vi "Buffer Num Readings.vi"(8 "error in (no error)":errorcluster, 9 "Buffer Name":string, 11 "VISA resource name":refnum<visa-resource-name>) -> (0 "error out":errorcluster, 1 "Number of Readings in Buffer":u32, 3 "VISA resource name out":refnum<visa-resource-name>, 4 "Command String":string)   [LabVIEW 2012, in "Keithley 2600 Series.lvlib"]
doc: "This VI queries the number of readings in the selected buffer.\n\n<b>Functions and Attributes Used</b>\n<buffername>.n"
uses:
  Keithley 2600 Series.lvlib
  Private/GlobalVariables.vi
panel:
  # "(c) 2008 Keithley Instruments, Inc.  ALL RIGHTS RESERVED."
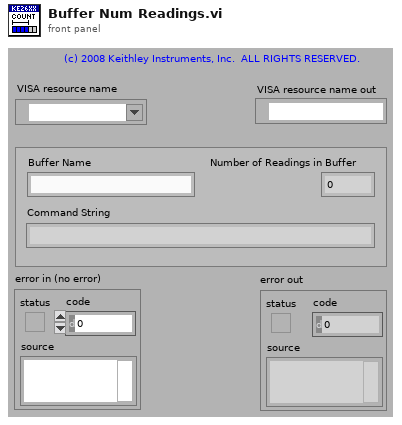
[diagram p1: front panel]
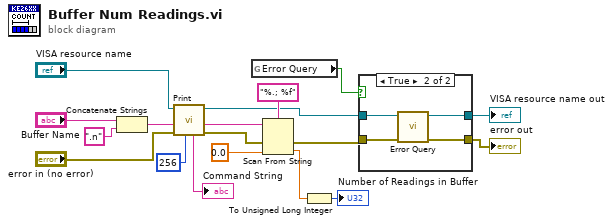
[diagram p0: block diagram]
diagram:
  n1 = Concatenate Strings("Buffer Name", ".n" ("string")) -> (w8:string)
  n2 = call "Print.vi"("Byte Count (1024)"=u32 256, "error in (no error)"="error in (no error)", "Input"=w8, "VISA resource name"="VISA resource name") -> ("error out"=w2:errorcluster, "Output"=w3:string, "VISA resource name out"=w1:refnum<visa-resource-name>, "Command String"=→"Command String":string)  [unwired: 1 in, 3 out]
  n3 = global read "GlobalVariables.vi" "Error Query"() -> (w14:bool)
  n4 = Scan From String(format string="%.; %f", input string=w3, error in=w2, default 1=0.0 ("default value 1")) -> (error out=w13:errorcluster, output 1=w15:dbl)  [unwired: 1 in, 2 out]
  n5 = To Unsigned Long Integer(number=w15) -> (unsigned 32bit integer=→"Number of Readings in Buffer":u32)
  n6 = case shown="True" w14 {
    tunnel: w13 -> [w20 w24]
    tunnel: [w19 w23] -> w12
    tunnel: [w20 w22] -> w11
    tunnel: w1 -> [w19 w21]
    frame False {
    }
    frame True {
      n7 = call "Error Query.vi"("error in (no error)"=w24, "VISA resource name"=w21) -> ("error out"=w22:errorcluster, "VISA resource name out"=w23:refnum<visa-resource-name>)  [unwired: 8 out]
    }
  }
  "VISA resource name out" <- w12
  "error out" <- w11
